vi "ResourceVisa_19version.vi"() -> ()   [LabVIEW 2019]
panel:
  out "display file":string
  in  "Path":path
  out "display m3510A":string
  in  "Voltmeter Picotest M3510A":refnum<visa-resource-name>
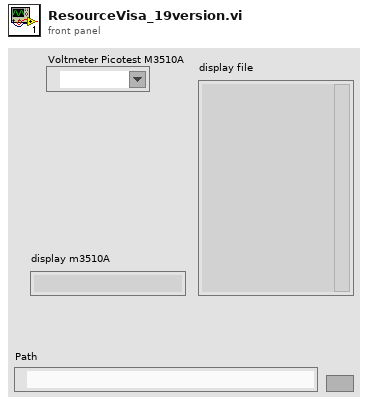
[diagram p1: front panel]
types:
  T1 = enum16{"read/write", "read-only", "write-only", ""}
  T2 = enum16{"open", "replace", "create", "open or create", "replace or create", "replace or create with confirmation", ""}
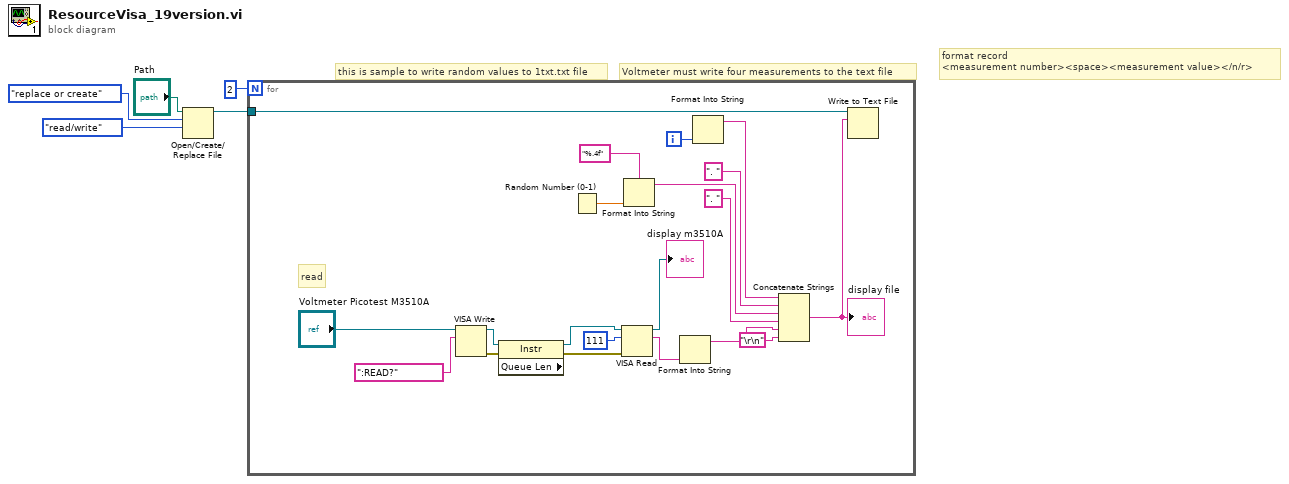
[diagram p0: block diagram]
diagram:
  # "format record \n<measurement number><space><measurement value></n/r>"
  # "Voltmeter must write four measurements to the text file"
  # "this is sample to write random values to 1txt.txt file"
  n1 = Open/Create/Replace File(file path (use dialog)="Path", operation (0:open)=T2."replace or create", access (0:read/write)=T1."read/write") -> (refnum out=w1:refnum<file>)  [unwired: 3 in, 2 out]
  n2 = for {
    N: 2 -> [_]
    tunnel: w1 -> [w17]
    i -> [w16]
    # "read"
    n3 = VISA Write(VISA resource name="Voltmeter Picotest M3510A", write buffer=":READ?") -> (VISA resource name out=w22:refnum<visa-resource-name>, error out=w23:errorcluster)  [unwired: 1 in, 1 out]
    n4 = property class="Instr" props=["Queue Len"](reference=w22, error in=w23) -> (reference out=w21:refnum<visa-resource-name>, error out=w20:errorcluster)  [unwired: 1 out]
    n5 = Random Number (0-1)() -> (number: 0 to 1=w18:dbl)
    n6 = VISA Read(VISA resource name=w21, byte count=111, error in (no error)=w20) -> (VISA resource name out=→"display m3510A":refnum<visa-resource-name>, read buffer=w6:string)  [unwired: 2 out]
    n7 = Format Into String(format string="%.4f", w18) -> (resulting string=w13:string)  [unwired: 2 in, 1 out]
    n8 = Format Into String(w6) -> (resulting string=w8:string)  [unwired: 3 in, 1 out]
    n9 = Format Into String(w16) -> (resulting string=w15:string)  [unwired: 3 in, 1 out]
    n10 = Concatenate Strings(w15, ". ", w13, ". ", w8, "\r\n") -> (w9:string)
    "display file" <- w9
    n11 = Write to Text File(file (use dialog)=w17, text=w9) -> ()  [unwired: 2 in, 3 out]
  }
